vi "Launch Root Panel core.vi"(6 "timeout in ms (-1)":i32=-1, 8 "Error In":errorcluster, 10 "Panel":refnum<class "Panel.lvclass">, 11 "Panel Actor in":refnum<class "Panel Actor.lvclass">) -> (0 "Error Out":errorcluster, 2 "Actor's Enqueuer":refnum<class "Message Enqueuer.lvclass">)   [LabVIEW 2019, in "Panel Actor.lvlib" / "Panel Actor.lvclass"]
doc: "Launches a Root Panel using any panel type.\n\n<B>Panel Actor In:</B> Panel Actor object to launch\n<B>Window Position:</B> Window Position object to control window position behavior.\n<B>timeout in ms</B> Time to wait for the panel to initialize\n<B>Error In:</B> Describes error conditions that occur before this node runs.\n\n<B>Actor's Enqueuer:</B> Enqueuer for newly spawned actor\n<B>Error Out:</B> Contains error information.\n\n----\nPlease see the following web address for additional documentation and tutorial information:\nhttp://www.mooregoodideas.com/mgi-panel-manager/\n\nAuthor: Derek Trepanier\n\nCopyright (c) 2018, Moore Good Ideas, Inc.\n\nAll rights reserved.\n\nRedistribution and use in source and binary forms, with or without modification, are permitted provided that the following conditions are met:\n\n * Redistributions of source code must retain the above copyright notice, this list of conditions and the following disclaimer.\n * Redistributions in binary form must reproduce the above copyright notice, this list of conditions and the following disclaimer in the documentation and/or other materials provided with the distribution.\n * Neither the name of Moore Good Ideas, Inc. nor the names of its contributors may be used to endorse or promote products derived from this software without specific prior written permission.\n\nTHIS SOFTWARE IS PROVIDED BY THE COPYRIGHT HOLDERS AND CONTRIBUTORS \"AS IS\" AND ANY EXPRESS OR IMPLIED WARRANTIES, INCLUDING, BUT NOT LIMITED TO, THE IMPLIED WARRANTIES OF MERCHANTABILITY AND FITNESS FOR A PARTICULAR PURPOSE ARE DISCLAIMED. IN NO EVENT SHALL THE COPYRIGHT OWNER OR CONTRIBUTORS BE LIABLE FOR ANY DIRECT, INDIRECT, INCIDENTAL, SPECIAL, EXEMPLARY, OR CONSEQUENTIAL DAMAGES (INCLUDING, BUT NOT LIMITED TO, PROCUREMENT OF SUBSTITUTE GOODS OR SERVICES; LOSS OF USE, DATA, OR PROFITS; OR BUSINESS INTERRUPTION) HOWEVER CAUSED AND ON ANY THEORY OF LIABILITY, WHETHER IN CONTRACT, STRICT LIABILITY, OR TORT (INCLUDING NEGLIGENCE OR OTHERWISE) ARISING IN ANY WAY OUT OF THE USE OF THIS SOFTWARE, EVEN IF ADVISED OF THE POSSIBILITY OF SUCH DAMAGE."
uses:
  Panel Actor.lvclass
  builds/Engine/Panel.lvlibp/Init Waiter/Init Waiter.lvclass
  builds/Engine/Panel.lvlibp/Panel/Panel.lvclass
  builds/Engine/Actor Framework.lvlibp/1abvi3w/vi.lib/ActorFramework/Actor/Actor.lvclass
  C:/Users/Public/Documents/Development/builds/Engine/Monitored Actor.lvlibp/Monitored Actor/Monitored Actor/Monitored Actor.lvclass
  C:/Users/Public/Documents/Development/builds/Engine/Engine.lvlibp/Project/Engine.lvclass
  C:/Users/Public/Documents/Development/builds/Engine/Actor Framework.lvlibp/1abvi3w/vi.lib/ActorFramework/Actor/Actor.lvclass
  builds/Engine/Actor Framework.lvlibp/1abvi3w/vi.lib/ActorFramework/Message Enqueuer/Message Enqueuer.lvclass
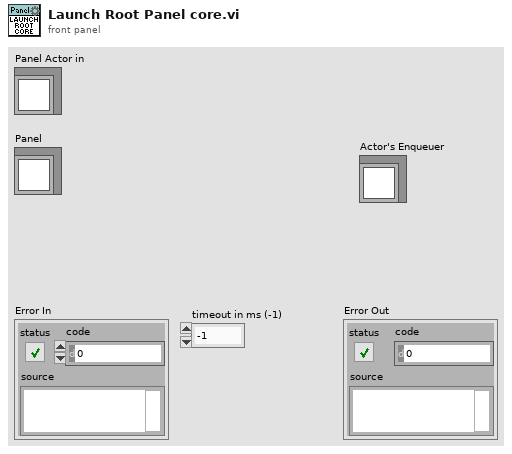
[diagram p1: front panel]
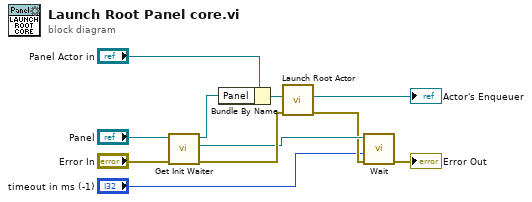
[diagram p0: block diagram]
diagram:
  n1 = call "Get Init Waiter.vi"("Error In"="Error In", "Panel In"="Panel") -> ("Error Out"=w6:errorcluster, "Init Waiter"=w5:refnum<class "Init Waiter.lvclass">, "Panel Out"=w1:refnum<class "Panel.lvclass">)  [unwired: 7 in]
  n2 = Bundle By Name(cluster="Panel Actor in", "Panel"=w1) -> (w10:refnum<class "Panel Actor.lvclass">)
  n3 = call "Launch Root Actor.vi"("error in (no error)"=w6, "Actor"=w10) -> ("error out"=w4:errorcluster, "Actor's Enqueuer"=→"Actor's Enqueuer":refnum<class "Message Enqueuer.lvclass">)  [unwired: 8 in]
  n4 = call "Wait.vi"("Error In"=w4, "timeout in ms (-1)"="timeout in ms (-1)", "Init Waiter in"=w5) -> ("Error Out"=→"Error Out":errorcluster)  [unwired: 7 in, 1 out]
